vi "Periodic Tasks.vi"(8 "error in":errorcluster) -> ()   [LabVIEW 2020]
doc: "This VI runs in parallel to other tasks. It can contain as many user-defined periodic loops as you need. These can carry out PID or other sorts of timed response."
uses:
  <vilib>/Rock Robotics/WPI/ThirdParty/REV Robotics/REVLib/Typedef/Spark MAX Idle Mode.ctl
  <vilib>/Rock Robotics/WPI/Utilities/WPI_GetSetVariantRefNum.vi
panel:
  out "Get Current Limit":dbl
  in  "Set Current Limit":sgl=100.0
  out "Get Ramp Rate":dbl
  in  "Set Ramp Rate":sgl
  out "Get Idle Mode":T1
  in  "Set Idle Mode":T1
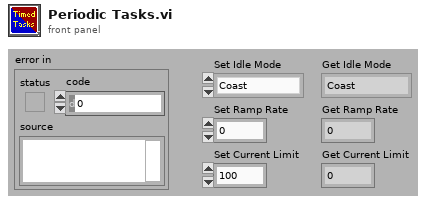
[diagram p1: front panel]
types:
  T1 = typedef "Spark MAX Idle Mode.ctl" = enum16{"Coast", "Brake"}
  T2 = typedef "WPI_JoystickDevRef.ctl" = cluster{"Device":T3}
  T3 = typedef "WPI_JoystickDeviceEnum.ctl" = enum16{"USB 0", "USB 1", "USB 2", "USB 3", "USB 4", "USB 5"}
  T4 = typedef "WPI_MotorControlDeviceRef.ctl" = cluster{"DeviceStatus":errorcluster, "Type":T5, "PWM":cluster{"PWM Channel":T6, "DeadBand":T7}, "CAN":cluster{"Device Number":u8, "SetOutput VI Ref":variant, "GetOutput VI Ref":variant, "Enable VI Ref":variant, "Disable VI Ref":variant, "Data":variant}, "Invert":bool, "DIO PWM":cluster{"PWM \"Enable\" Channel":T6, "DIOChannel":T8, "PWM Rate":dbl}}
  T5 = typedef "WPI_MotorControlType.ctl" = enum16{"PWM", "CAN", "DIO PWM"}
  T6 = typedef "FPGA_DIOPWMChannel.ctl" = enum8{"PWM 0", "PWM 1", "PWM 2", "PWM 3", "PWM 4", "PWM 5", "PWM 6", "PWM 7", "PWM 8", "PWM 9", "PWM MXP 0", "PWM MXP 1", "PWM MXP 2", "PWM MXP 3", "PWM MXP 4", "PWM MXP 5", "PWM MXP 6", "PWM MXP 7", "PWM MXP 8", "PWM MXP 9", "Invalid"}
  T7 = typedef "WPI_PWMDeadband.ctl" = cluster{"Name":string, "maxPositivePwm":i32, "minPositivePwm":i32, "centerPwm":i32, "maxNegativePwm":i32, "minNegativePwm":i32, "angularRange":u16}
  T8 = typedef "FPGA_DIOChannel.ctl" = enum8{"DIO 0", "DIO 1", "DIO 2", "DIO 3", "DIO 4", "DIO 5", "DIO 6", "DIO 7", "DIO 8", "DIO 9", "DIO MXP 0", "DIO MXP 1", "DIO MXP 2", "DIO MXP 3", "DIO MXP 4", "DIO MXP 5", "DIO MXP 6", "DIO MXP 7", "DIO MXP 8", "DIO MXP 9", "DIO MXP 10", "DIO MXP 11", "DIO MXP 12", "DIO MXP 13", "DIO MXP 14", "DIO MXP 15", "SPI Port CS1", "SPI Port CS2", "SPI Port CS3", "SPI Port MISO", "SPI Port MOSI", "Invalid"}
  T9 = cluster{"JoystickDevRef":T2, "MotorControlDevRef":T4}
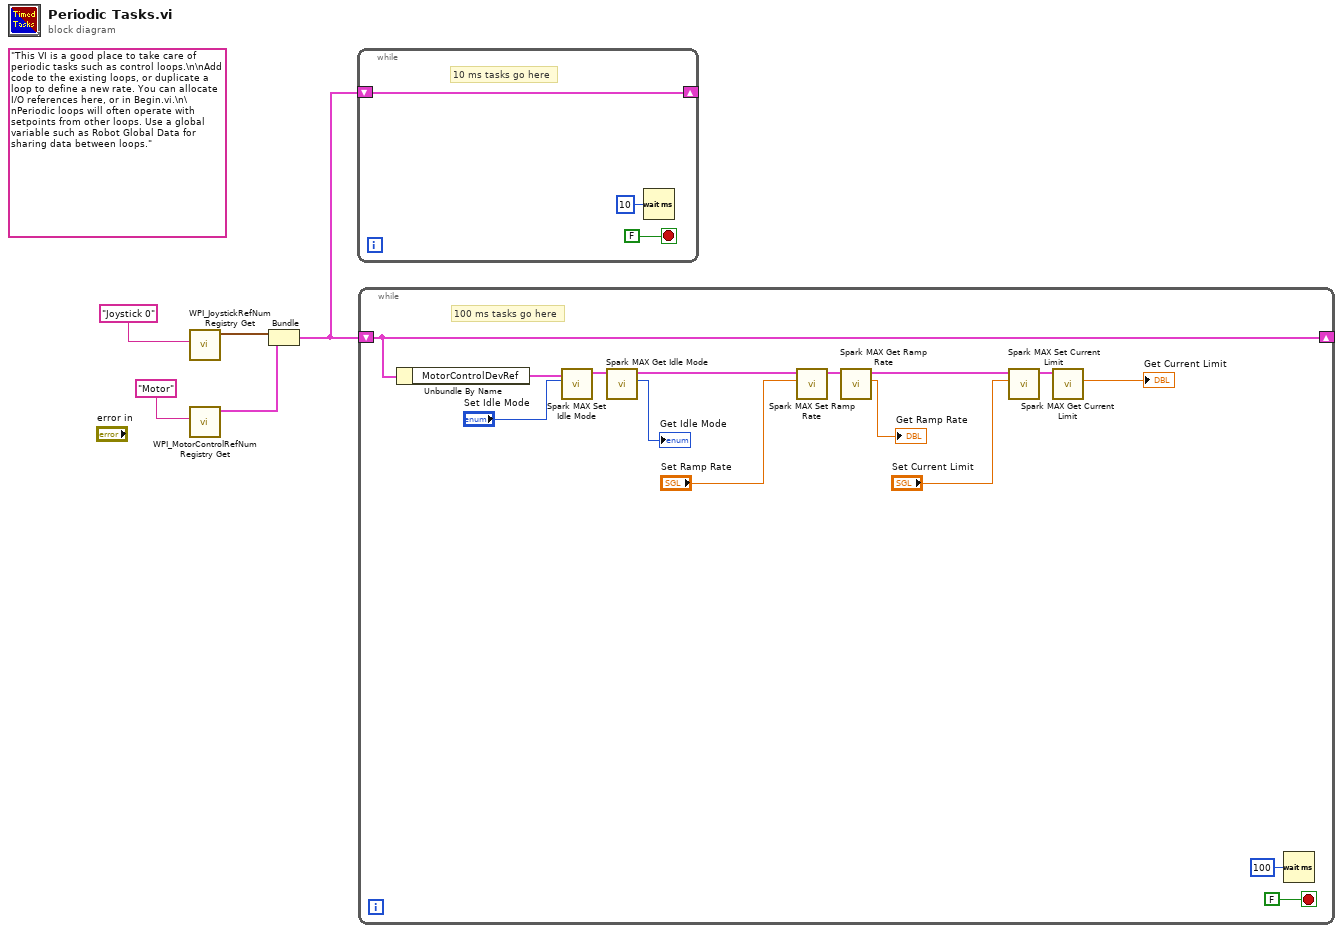
[diagram p0: block diagram]
diagram:
  (unwired) "This VI is a good place to take care of periodic tasks such as control loops.\n\nAdd code to the existing loops, or duplicate a loop to define a new rate. You can allocate I/O references here, or in Begin.vi.\n\nPeriodic loops will often operate with setpoints from other loops. Use a global variable such as Robot Global Data for sharing data between loops."
  n1 = call <vilib>:"WPI_JoystickRefNum Registry Get.vi"("refnum name"="Joystick 0") -> ("JoystickDevRef"=w3:T2)  [unwired: 1 in, 9 out]
  n2 = call <vilib>:"WPI_MotorControlRefNum Registry Get.vi"("refnum name"="Motor") -> ("MotorControlDevRef"=w2:T4)  [unwired: 9 in, 1 out]
  n3 = Bundle("JoystickDevRef"=w3, "MotorControlDevRef"=w2) -> (w1:T9)  [unwired: 1 out]
  n4 = while {
    shift-right: [w6] -> _
    shift-left: w1 -> [w6]
    stop <- FALSE stop-if-true
    # "10 ms tasks go here"
    n5 = Wait (ms)(milliseconds to wait=u32 10) -> ()  [unwired: 1 out]
  }
  n6 = while {
    shift-right: [w21] -> _
    shift-left: w1 -> [w21]
    stop <- FALSE stop-if-true
    # "100 ms tasks go here"
    n7 = Unbundle By Name(w21) -> ("MotorControlDevRef"=w20:T4)
    n8 = call <vilib>:"Spark MAX Set Idle Mode.vi"("Idle Mode"="Set Idle Mode", "MotorControlDeviceRef in"=w20) -> ("MotorControlDeviceRef out"=w18:T4)  [unwired: 8 in, 1 out]
    n9 = call <vilib>:"Spark MAX Get Idle Mode.vi"("MotorControlDeviceRef in"=w18) -> ("Idle Mode"=→"Get Idle Mode":T1, "MotorControlDeviceRef out"=w16:T4)  [unwired: 8 in, 1 out]
    n10 = call <vilib>:"Spark MAX Set Ramp Rate.vi"("Seconds from neutral to full (0)"="Set Ramp Rate", "MotorControlDeviceRef in"=w16) -> ("MotorControlDeviceRef"=w14:T4)  [unwired: 8 in, 1 out]
    n11 = call <vilib>:"Spark MAX Get Ramp Rate.vi"("MotorControlDeviceRef in"=w14) -> ("Ramp Rate"=→"Get Ramp Rate":dbl, "MotorControlDeviceRef out"=w12:T4)  [unwired: 8 in, 1 out]
    n12 = call <vilib>:"Spark MAX Set Current Limit.vi"("Current Limit A (100)"="Set Current Limit", "MotorControlDeviceRef in"=w12) -> ("MotorControlDeviceRef out"=w10:T4)  [unwired: 8 in, 1 out]
    n13 = call <vilib>:"Spark MAX Get Current Limit.vi"("MotorControlDeviceRef in"=w10) -> ("Current Limit"=→"Get Current Limit":dbl)  [unwired: 7 in, 3 out]
    n14 = Wait (ms)(milliseconds to wait=u32 100) -> ()  [unwired: 1 out]
  }
